vi "rs3 delete sensor.vi"(8 "error in (no error)":errorcluster, 11 "sensor":u64) -> (0 "error out":errorcluster, 3 "error":u64)   [LabVIEW 2019, in "libRealSense3.lvlib"]
doc: "Delete the SENSOR after it has been stopped and closed."
uses:
  libRealSense3.lvlib
  realsense2.dll
panel:
  # "RS3 Delete Sensor"
  # "(C) Intel Corp. 2017,  AGJ"
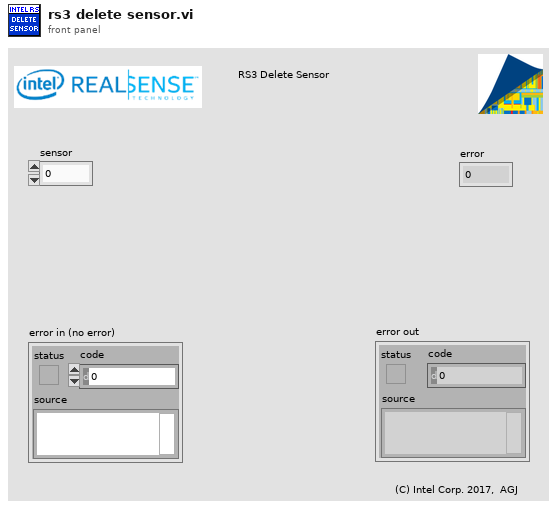
[diagram p1: front panel]
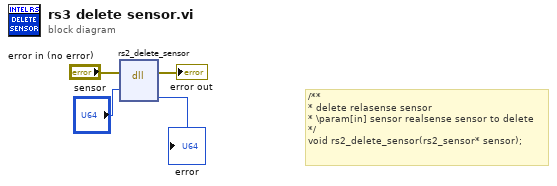
[diagram p0: block diagram]
diagram:
  # "/**\n* delete relasense sensor\n* \\param[in] sensor realsense sensor to delete\n*/\nvoid rs2_delete_sensor(rs2_sensor* sensor);"
  n1 = dll-call lib="C:/Users/morte/Documents/gitmoro/treadmill/RealSense for Labview ver. 2.33/realsense2.dll" fn="rs2_delete_sensor"(error in="error in (no error)", "sensor"="sensor") -> (error out=→"error out":errorcluster, "error"=→"error":u64)  [unwired: 5 in, 1 out]
